vi "Construct Limit Comparison Option List.vi"(9 "Hidden?":bool, 10 "ID":string, 11 "Comparison":T1) -> (3 "String":string)   [LabVIEW 2011]
uses:
  PI Limit Comparison.ctl
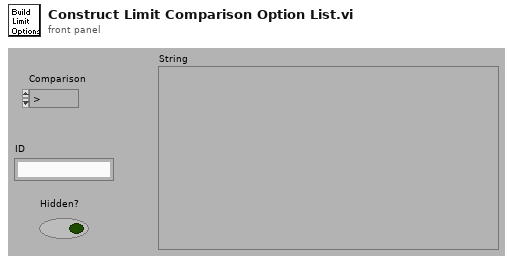
[diagram p1: front panel]
types:
  T1 = typedef "PI Limit Comparison.ctl" = enum16{">", ">=", "<", "<=", "<>", "="}
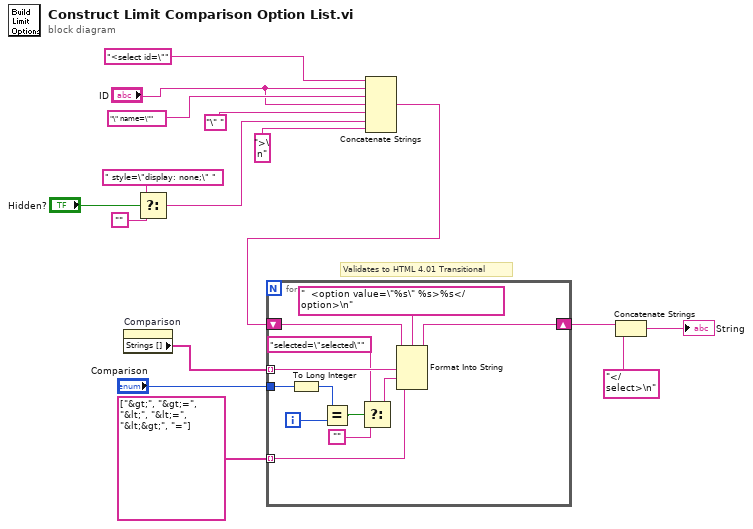
[diagram p0: block diagram]
diagram:
  # "Validates to HTML 4.01 Transitional"
  n1 = property on="Comparison" class="Enum (strict)"() -> ("Strings []"=w6:string[])  [unwired: 2 in, 2 out]
  n2 = Select(t=" style=\"display: none;\" ", s="Hidden?", f="") -> (s? t:f=w10:string)
  n3 = Concatenate Strings("<select id=\"", "ID", "\" name=\"", "ID", "\" ", w10, ">\n") -> (w4:string)
  n4 = for {
    shift-right: [w26] -> w2
    shift-left: w4 -> [w28]
    tunnel: "Comparison" -> [w18]
    tunnel: w6 -> [w24] mode=indexing
    tunnel: string[] ["&gt;", "&gt;=", "&lt;", "&lt;=", "&lt;&gt;", "="] -> [w21] mode=indexing
    i -> [w25]
    n5 = To Long Integer(number=w18) -> (32bit integer=w17:i32)
    n6 = Equal?(x=w17, y=w25) -> (x = y?=w23:bool)
    n7 = Select(t="selected=\"selected\"", s=w23, f="") -> (s? t:f=w20:string)
    n8 = Format Into String(format string="  <option value=\"%s\" %s>%s</option>\n", initial string=w28, w24, w20, w21) -> (resulting string=w26:string)  [unwired: 1 in, 1 out]
  }
  n9 = Concatenate Strings(w2, "</select>\n") -> (→"String":string)
